vi "Move XYZ.vi"(0 "PID Gains In":T1={"X PID"={"proportional gain (Kc)"=0.03, "integral time (Ti, min)"=0.0, "derivative time (Td, min)"=0.0}, "Y PID"={"proportional gain (Kc)"=0.03, "integral time (Ti, min)"=0.0, "derivative time (Td, min)"=0.0}, "Z PID"={"proportional gain (Kc)"=0.035, "integral time (Ti, min)"=0.0, "derivative time (Td, min)"=0.0}} {"Z PID"."derivative time (Td, min)" format="%.3f"; "Z PID"."integral time (Ti, min)" format="%.3f"; "Z PID"."proportional gain (Kc)" format="%.3f"; "Y PID"."derivative time (Td, min)" format="%.3f"; "Y PID"."integral time (Ti, min)" format="%.3f"; "Y PID"."proportional gain (Kc)" format="%.3f"; "X PID"."derivative time (Td, min)" format="%.3f"; "X PID"."integral time (Ti, min)" format="%.3f"; "X PID"."proportional gain (Kc)" format="%.3f"}, 5 "Y Target":dbl, 6 "X Target":dbl, 10 "Max Time":dbl=90.0, 11 "Gyro Target":dbl=-180.0, 12 "Movement":dbl=3.0, 14 "X Output Range":cluster{"output high":dbl, "output low":dbl}={"output high"=0.8, "output low"=-0.8}, 15 "X Stop Threshold":dbl=5.0, 16 "Y Output Range":cluster{"output high":dbl, "output low":dbl}={"output high"=0.8, "output low"=-0.8}, 17 "Y Stop Threshold":dbl=5.0, 18 "Z Output Range":cluster{"output high":dbl, "output low":dbl}={"output high"=0.8, "output low"=-0.8}, 19 "Z  Stop Threshold":dbl=8.0) -> ()   [LabVIEW 2018]
uses:
  Robot Global Data.vi
  SubSystems/Drive Train/Drive Train Global.vi
  SubSystems/Hatch Panel Intake/Hatch Panel Intake Global.vi
  SubSystems/Lift/Lift Global.vi
  <vilib>/addons/control/pid/pid.llb/PID (DBL).vi
  <vilib>/addons/control/pid/NI_PID_pid.lvlib
panel:
  in  "Minimum Time":u32=500
  in  "Settle Time":u32=2000
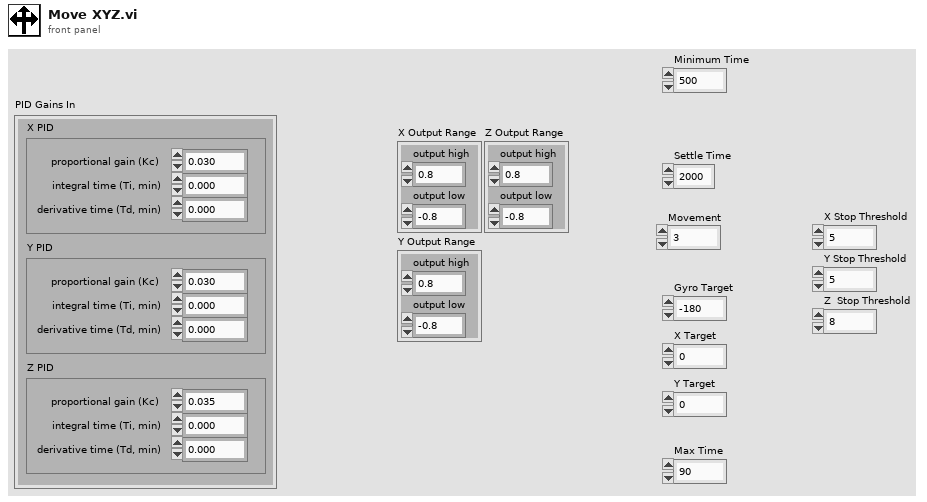
[diagram p1: front panel]
types:
  T1 = cluster{"X PID":cluster{"proportional gain (Kc)":dbl, "integral time (Ti, min)":dbl, "derivative time (Td, min)":dbl}, "Y PID":cluster{"proportional gain (Kc)":dbl, "integral time (Ti, min)":dbl, "derivative time (Td, min)":dbl}, "Z PID":cluster{"proportional gain (Kc)":dbl, "integral time (Ti, min)":dbl, "derivative time (Td, min)":dbl}}
  T2 = cluster{"proportional gain (Kc)":dbl, "integral time (Ti, min)":dbl, "derivative time (Td, min)":dbl}
  T3 = cluster{"Rollover":dbl, "Yaw":dbl, "Cont Yaw":dbl}
  T4 = cluster{"offsetAngle H":dbl, "offsetAngle V":dbl, "area":dbl, "skew":dbl, "validTarget":dbl, "latency":dbl}
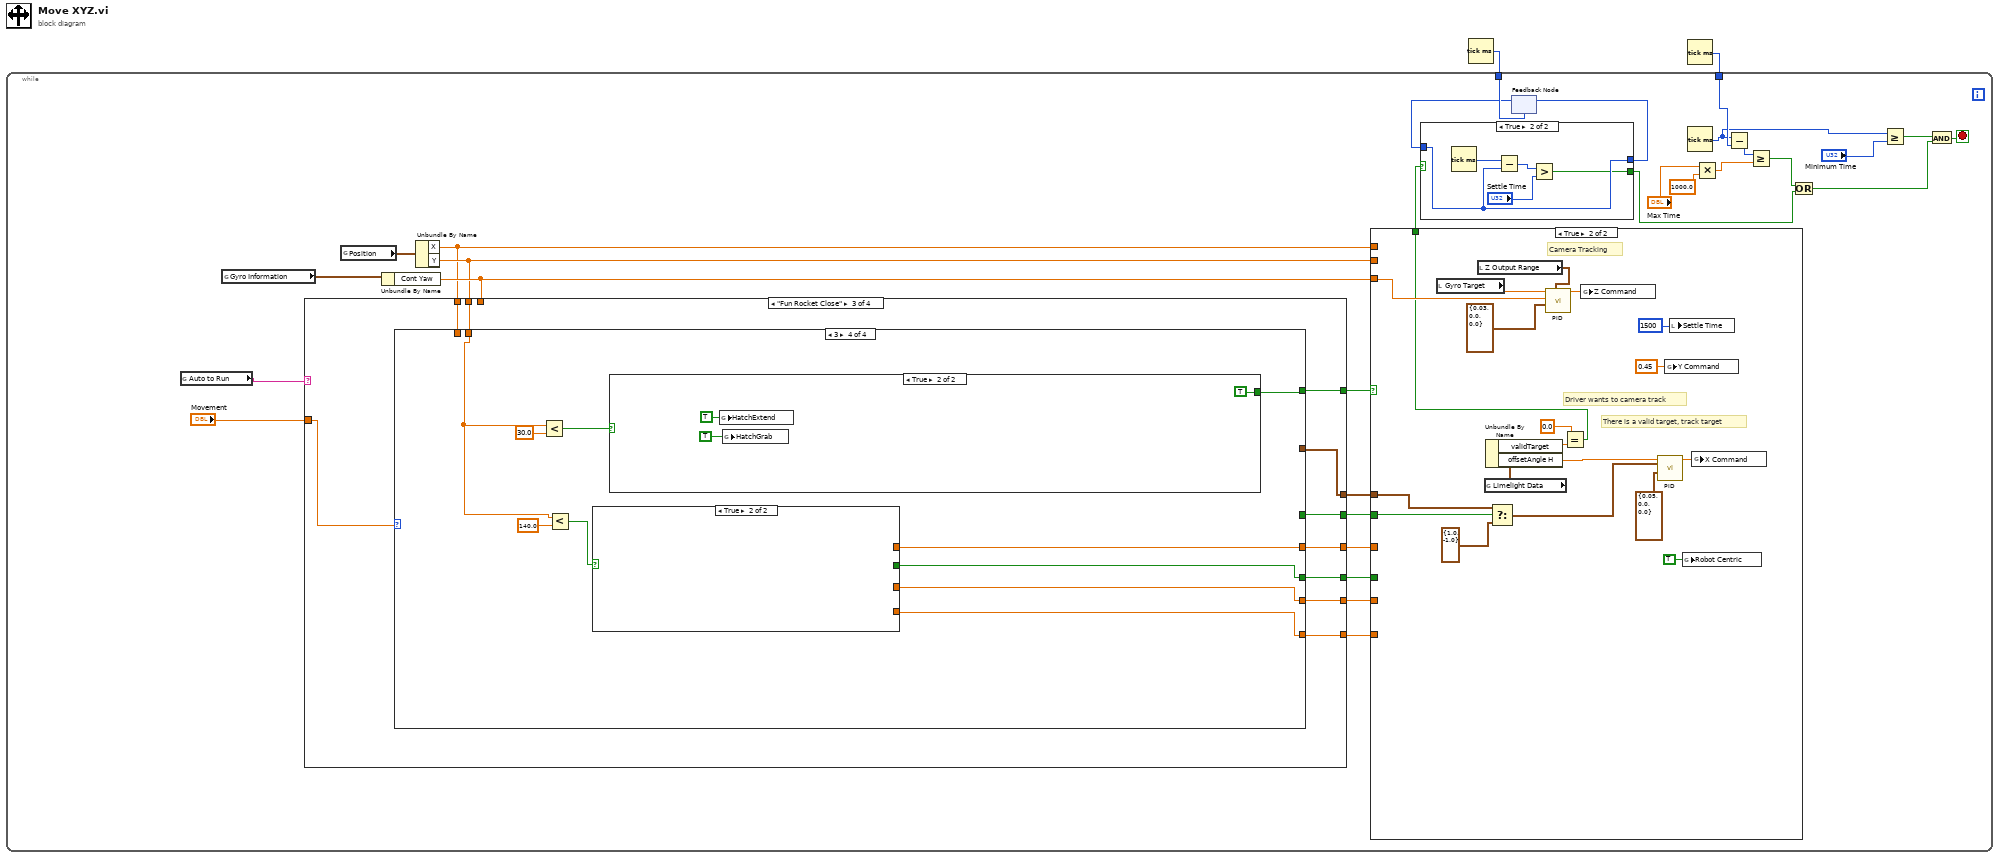
[diagram p0: block diagram]
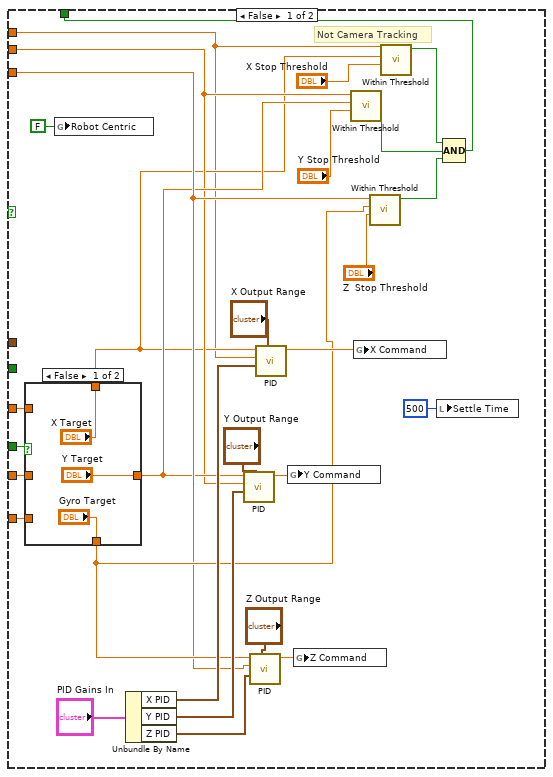
[diagram p2: hidden frame]
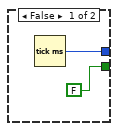
[diagram p4: hidden frame]
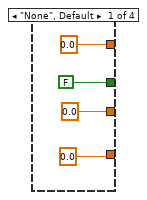
[diagram p5: hidden frame]
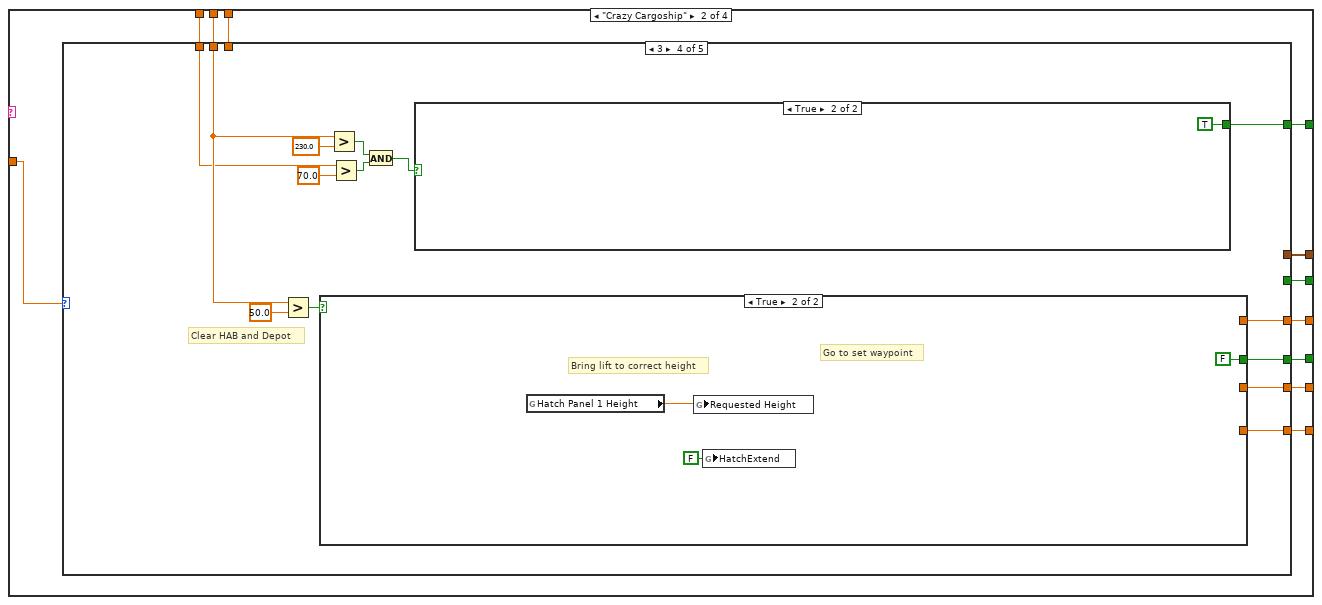
[diagram p6: hidden frame]
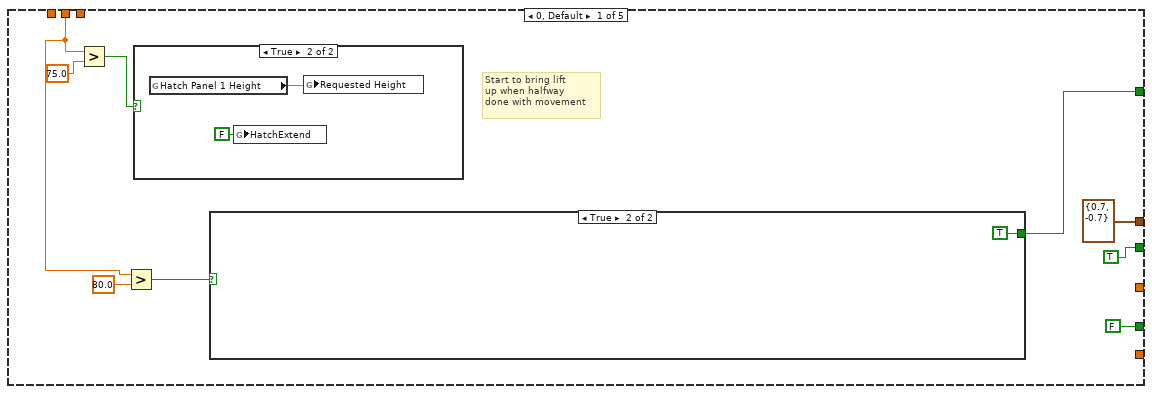
[diagram p7: hidden frame]
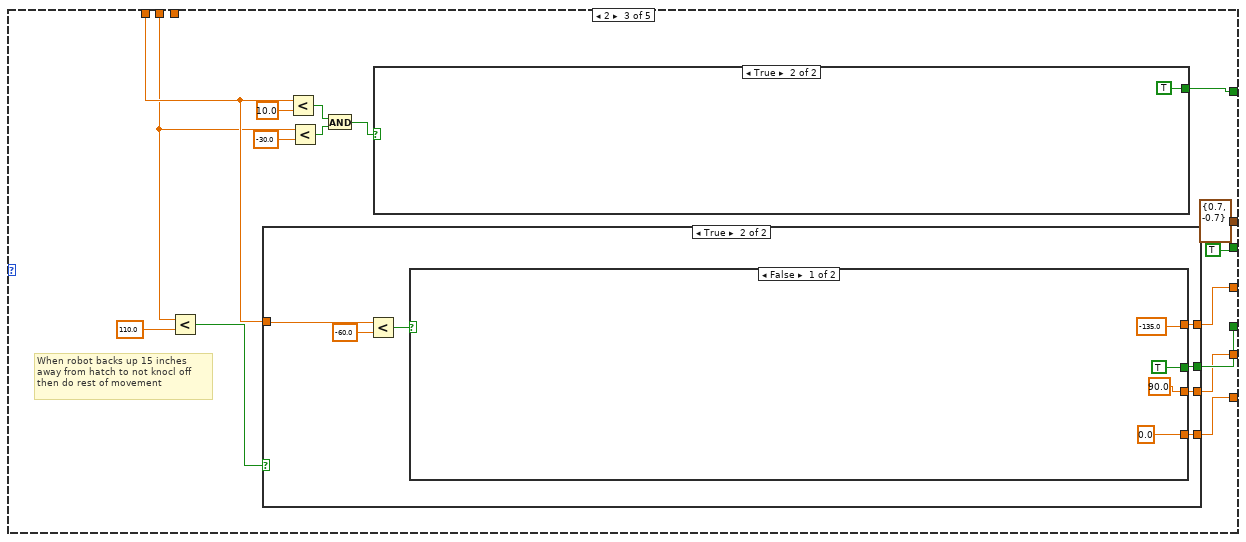
[diagram p11: hidden frame]
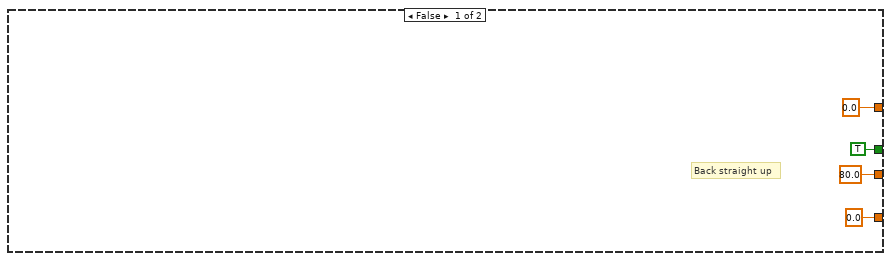
[diagram p13: hidden frame]
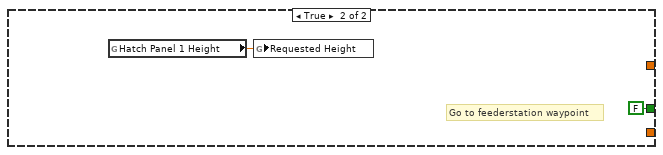
[diagram p14: hidden frame]
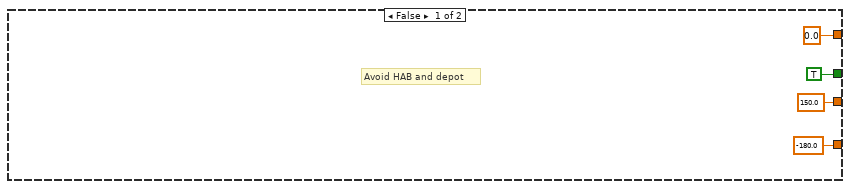
[diagram p16: hidden frame]
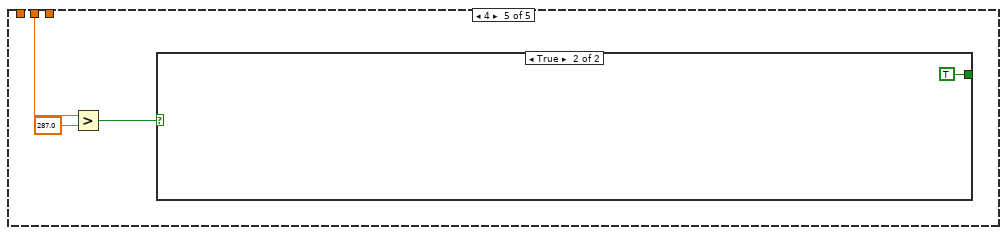
[diagram p17: hidden frame]
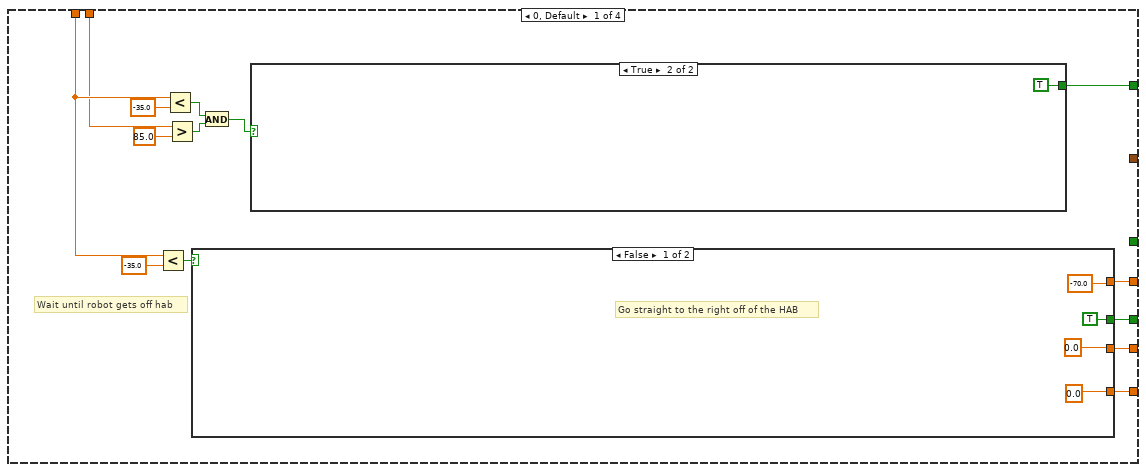
[diagram p19: hidden frame]
diagram:
  n1 = Tick Count (ms)() -> (millisecond timer value=w2:u32)
  n2 = Tick Count (ms)() -> (millisecond timer value=w1:u32)
  n3 = while {
    tunnel: w2 -> [w26]
    tunnel: w1 -> [w11]
    stop <- w10 stop-if-true
    n4 = global read "Robot Global Data.vi" "Auto to Run"() -> (w23:string)
    n5 = global read "Drive Train Global.vi" "Gyro Information"() -> (w20:T3)
    n6 = global read "Drive Train Global.vi" "Position"() -> (w22:cluster{"X":dbl, "Y":dbl})
    n7 = Unbundle By Name(w20) -> ("Cont Yaw"=w18:dbl)
    n8 = Unbundle By Name(w22) -> ("X"=w16:dbl, "Y"=w17:dbl)
    n9 = case shown="\"Fun Rocket Close\"" w23 {
      tunnel: [0.0 w103 w186 w268] -> w32
      tunnel: [0.0 w102 w185 w267] -> w31
      tunnel: [0.0 w101 w184 w266] -> w30
      tunnel: w17 -> [_ w107 w189 w271]
      tunnel: [FALSE w106 w187 w269] -> w29
      tunnel: w16 -> [_ w104 w188 w270]
      tunnel: "Movement" -> [_ w108 w190 w272]
      tunnel: w18 -> [_ w105 _ w264]
      tunnel: [_ w100 w183 w265] -> w5
      tunnel: [_ w98 w181 _] -> w4
      tunnel: [_ w99 w182 _] -> w3
      frame "None", Default {
      }
      frame "Crazy Cargoship" {
        n10 = case shown="3" w108 {
          tunnel: w107 -> [w111 _ w123 w156 w177]
          tunnel: [FALSE _ w134 w168 _] -> w106
          tunnel: w105 -> [_ _ _ _ _]
          tunnel: w104 -> [_ _ w124 w155 _]
          tunnel: [_ _ w133 w165 _] -> w103
          tunnel: [_ _ w132 w164 _] -> w102
          tunnel: [_ _ w131 w163 _] -> w101
          tunnel: [w113 _ w125 w157 _] -> w100
          tunnel: [TRUE ("Robot Centric") _ TRUE ("Robot Centric") _ _] -> w99
          tunnel: [cluster{"output high":dbl, "output low":dbl} {"output high"=0.7, "output low"=-0.7} ("output range") _ cluster{"output high":dbl, "output low":dbl} {"output high"=0.7, "output low"=-0.7} ("output range") _ _] -> w98
          frame 0, Default {
            # "Start to bring lift\nup when halfway\ndone with movement"
            n11 = Greater?(x=w111, y=75.0) -> (0:w116:bool)
            n12 = Greater?(x=w111, y=80.0) -> (0:w112:bool)
            n13 = case shown="True" w116 {
              frame False {
              }
              frame True {
                n14 = global read "Lift Global.vi" "Hatch Panel 1 Height"() -> (w120:dbl)
                n15 = global write "Hatch Panel Intake Global.vi" "HatchExtend"(FALSE ("HatchGrab")) -> ()
                n16 = global write "Lift Global.vi" "Requested Height"(w120) -> ()
              }
            }
            n17 = case shown="True" w112 {
              tunnel: [_ TRUE] -> w113
              frame False {
              }
              frame True {
              }
            }
          }
          frame 1 {
          }
          frame 2 {
            # "When robot backs up 15 inches\naway from hatch to not knocl off\nthen do rest of movement"
            n18 = Less?(x=w123, y=110.0) -> (x < y?=w136:bool)
            n19 = case shown="True" w136 {
              tunnel: [TRUE w148] -> w134
              tunnel: [0.0 w144] -> w133
              tunnel: [80.0 w143] -> w132
              tunnel: [0.0 w142] -> w131
              tunnel: w124 -> [_ w145]
              frame False {
                # "Back straight up"
              }
              frame True {
                n20 = Less?(x=w145, y=-60.0) -> (x < y?=w146:bool)
                n21 = case shown="False" w146 {
                  tunnel: [TRUE FALSE] -> w148
                  tunnel: [-135.0 _] -> w144
                  tunnel: [90.0 _] -> w143
                  tunnel: [0.0 _] -> w142
                  frame False {
                  }
                  frame True {
                    # "Go to feederstation waypoint"
                    n22 = global read "Lift Global.vi" "Hatch Panel 1 Height"() -> (w153:dbl)
                    n23 = global write "Lift Global.vi" "Requested Height"(w153) -> ()
                  }
                }
              }
            }
            n24 = Less?(x=w124, y=10.0) -> (x < y?=w128:bool)
            n25 = Less?(x=w123, y=-30.0) -> (x < y?=w127:bool)
            n26 = And(x=w128, y=w127) -> (x .and. y?=w126:bool)
            n27 = case shown="True" w126 {
              tunnel: [_ TRUE] -> w125
              frame False {
              }
              frame True {
              }
            }
          }
          frame 3 {
            # "Clear HAB and Depot"
            n28 = Greater?(x=w156, y=50.0) -> (0:w167:bool)
            n29 = case shown="True" w167 {
              tunnel: [TRUE FALSE] -> w168
              tunnel: [0.0 _] -> w165
              tunnel: [150.0 _] -> w164
              tunnel: [-180.0 _] -> w163
              frame False {
                # "Avoid HAB and depot"
              }
              frame True {
                # "Bring lift to correct height"
                # "Go to set waypoint"
                n30 = global read "Lift Global.vi" "Hatch Panel 1 Height"() -> (w175:dbl)
                n31 = global write "Lift Global.vi" "Requested Height"(w175) -> ()
                n32 = global write "Hatch Panel Intake Global.vi" "HatchExtend"(FALSE ("HatchGrab")) -> ()
              }
            }
            n33 = Greater?(x=w156, y=230.0) -> (0:w160:bool)
            n34 = Greater?(x=w155, y=70.0) -> (0:w159:bool)
            n35 = And(x=w160, y=w159) -> (x .and. y?=w158:bool)
            n36 = case shown="True" w158 {
              tunnel: [_ TRUE] -> w157
              frame False {
              }
              frame True {
              }
            }
          }
          frame 4 {
            n37 = Greater?(x=w177, y=287.0) -> (0:w178:bool)
            n38 = case shown="True" w178 {
              tunnel: [_ TRUE] -> _
              frame False {
              }
              frame True {
              }
            }
          }
        }
      }
      frame "Fun Rocket Close" {
        n39 = case shown="3" w190 {
          tunnel: w189 -> [w197 w212 w231 w252]
          tunnel: w188 -> [w198 w217 _ _]
          tunnel: [w202 _ w229 w247] -> w187
          tunnel: [w201 _ w230 w250] -> w186
          tunnel: [w200 _ w228 w249] -> w185
          tunnel: [w199 _ w227 w248] -> w184
          tunnel: [w191 w218 w237 w255] -> w183
          tunnel: [_ _ w235 _] -> w182
          tunnel: [_ _ w234 _] -> w181
          frame 0, Default {
            # "Wait until robot gets off hab"
            n40 = Less?(x=w198, y=-35.0) -> (x < y?=w204:bool)
            n41 = Less?(x=w198, y=-35.0) -> (x < y?=w194:bool)
            n42 = Greater?(x=w197, y=85.0) -> (0:w193:bool)
            n43 = case shown="False" w204 {
              tunnel: [TRUE FALSE] -> w202
              tunnel: [-70.0 _] -> w201
              tunnel: [0.0 _] -> w200
              tunnel: [0.0 _] -> w199
              frame False {
                # "Go straight to the right off of the HAB"
              }
              frame True {
                # "Bring the lift up to the correct level because its slow"
                # "Robot off of HAB, go to the rocket"
                n44 = global read "Lift Global.vi" "Hatch Panel 2 Height"() -> (w210:dbl)
                n45 = global write "Lift Global.vi" "Requested Height"(w210) -> ()
              }
            }
            n46 = And(x=w194, y=w193) -> (x .and. y?=w192:bool)
            n47 = case shown="True" w192 {
              tunnel: [_ TRUE] -> w191
              frame False {
              }
              frame True {
              }
            }
          }
          frame 1 {
            n48 = Less?(x=w212, y=-17.0) -> (x < y?=w221:bool)
            n49 = Less?(x=w217, y=-90.0) -> (x < y?=w220:bool)
            n50 = Less?(x=w212, y=0.0) -> (x < y?=w215:bool)
            n51 = Less?(x=w212, y=-5.0) -> (x < y?=w214:bool)
            n52 = And(x=w221, y=w220) -> (x .and. y?=w219:bool)
            n53 = case shown="True" w215 {
              frame False {
              }
              frame True {
                n54 = global write "Hatch Panel Intake Global.vi" "HatchExtend"(TRUE ("HatchExtend")) -> ()
              }
            }
            n55 = case shown="True" w214 {
              frame False {
              }
              frame True {
                n56 = global write "Hatch Panel Intake Global.vi" "HatchGrab"(TRUE ("HatchExtend")) -> ()
              }
            }
            n57 = case shown="True" w219 {
              tunnel: [_ TRUE] -> w218
              frame False {
              }
              frame True {
              }
            }
          }
          frame 2 {
            # "back up then turn"
            n58 = Greater?(x=w231, y=150.0) -> (0:w236:bool)
            n59 = Greater?(x=w231, y=40.0) -> (0:w232:bool)
            n60 = case shown="True" w236 {
              tunnel: [_ TRUE] -> w237
              tunnel: [_ TRUE] -> w235
              tunnel: [_ cluster{"output high":dbl, "output low":dbl} {"output high"=0.6, "output low"=-0.6} ("output range")] -> w234
              frame False {
              }
              frame True {
              }
            }
            n61 = case shown="False" w232 {
              tunnel: [0.0 _] -> w230
              tunnel: [TRUE FALSE] -> w229
              tunnel: [200.0 _] -> w228
              tunnel: [-180.0 _] -> w227
              frame False {
              }
              frame True {
              }
            }
          }
          frame 3 {
            n62 = Less?(x=w252, y=30.0) -> (x < y?=w254:bool)
            n63 = Less?(x=w252, y=140.0) -> (x < y?=w251:bool)
            n64 = case shown="True" w251 {
              tunnel: [0.0 _] -> w250
              tunnel: [100.0 _] -> w249
              tunnel: [-30.0 _] -> w248
              tunnel: [TRUE _] -> w247
              frame False {
              }
              frame True {
              }
            }
            n65 = case shown="True" w254 {
              tunnel: [_ TRUE] -> w255
              frame False {
              }
              frame True {
                n66 = global write "Hatch Panel Intake Global.vi" "HatchExtend"(TRUE ("HatchExtend")) -> ()
                n67 = global write "Hatch Panel Intake Global.vi" "HatchGrab"(TRUE ("HatchExtend")) -> ()
              }
            }
          }
        }
      }
      frame "Fun Rocket Far" {
        n68 = case shown="2" w272 {
          tunnel: w271 -> [w275 w309 w328 w344]
          tunnel: w270 -> [w274 w307 _ _]
          tunnel: [w279 w305 w333 w339] -> w269
          tunnel: [w278 w306 w332 w342] -> w268
          tunnel: [w277 w304 w331 w341] -> w267
          tunnel: [w276 w303 w330 w340] -> w266
          tunnel: [w273 w312 _ w347] -> w265
          tunnel: w264 -> [_ _ _ _]
          frame 0, Default {
            # "Wait until robot gets off hab"
            n69 = Greater?(x=w275, y=160.0) -> (0:w281:bool)
            n70 = case shown="True" w281 {
              tunnel: [TRUE w294] -> w279
              tunnel: [-10.0 w292] -> w278
              tunnel: [170.0 w291] -> w277
              tunnel: [0.0 w290] -> w276
              tunnel: w274 -> [_ w287]
              tunnel: [_ w286] -> w273
              frame False {
              }
              frame True {
                # "Bring the lift up to the correct level because its slow"
                n71 = global read "Lift Global.vi" "Hatch Panel 2 Height"() -> (w293:dbl)
                n72 = global write "Lift Global.vi" "Requested Height"(w293) -> ()
                n73 = Less?(x=w287, y=-60.0) -> (x < y?=w288:bool)
                n74 = case shown="False" w288 {
                  tunnel: [TRUE FALSE] -> w294
                  tunnel: [-100.0 ("y") _] -> w292
                  tunnel: [195.0 ("y") _] -> w291
                  tunnel: [-150.0 ("y") _] -> w290
                  tunnel: [_ TRUE] -> w286
                  frame False {
                  }
                  frame True {
                  }
                }
              }
            }
          }
          frame 1 {
            n75 = Less?(x=w309, y=-30.0) -> (x < y?=w315:bool)
            n76 = Greater?(x=w307, y=65.0) -> (0:w314:bool)
            n77 = Less?(x=w309, y=0.0) -> (x < y?=w310:bool)
            n78 = And(x=w315, y=w314) -> (x .and. y?=w313:bool)
            n79 = case shown="True" w310 {
              frame False {
              }
              frame True {
                n80 = global write "Hatch Panel Intake Global.vi" "HatchExtend"(TRUE ("HatchExtend")) -> ()
                n81 = global write "Hatch Panel Intake Global.vi" "HatchGrab"(TRUE ("HatchExtend")) -> ()
              }
            }
            n82 = Greater?(x=w307, y=-40.0) -> (0:w301:bool)
            n83 = case shown="False" w313 {
              tunnel: [FALSE TRUE] -> w312
              frame False {
              }
              frame True {
              }
            }
            n84 = call "Flip Flop.vi"("Line 1"=w301) -> ("Switch"=w302:bool)  [unwired: 10 in]
            n85 = case shown="True" w302 {
              tunnel: [_ -30.0 ("y")] -> w306
              tunnel: [FALSE TRUE] -> w305
              tunnel: [_ 190.0 ("y")] -> w304
              tunnel: [_ -150.0 ("y")] -> w303
              frame False {
              }
              frame True {
              }
            }
          }
          frame 2 {
            n86 = Less?(x=w328, y=30.0) -> (x < y?=w329:bool)
            n87 = case shown="False" w329 {
              tunnel: [TRUE FALSE] -> w333
              tunnel: [-30.0 _] -> w332
              tunnel: [100.0 _] -> w331
              tunnel: [-180.0 _] -> w330
              frame False {
              }
              frame True {
              }
            }
          }
          frame 3 {
            n88 = Less?(x=w344, y=30.0) -> (x < y?=w346:bool)
            n89 = Less?(x=w344, y=140.0) -> (x < y?=w343:bool)
            n90 = case shown="False" w343 {
              tunnel: [0.0 _] -> w342
              tunnel: [100.0 _] -> w341
              tunnel: [-30.0 _] -> w340
              tunnel: [TRUE _] -> w339
              frame False {
              }
              frame True {
              }
            }
            n91 = case shown="True" w346 {
              tunnel: [_ TRUE] -> w347
              frame False {
              }
              frame True {
              }
            }
          }
        }
      }
    }
    n92 = case shown="True" w5 {
      tunnel: w32 -> [w54 _]
      tunnel: w31 -> [w53 _]
      tunnel: w30 -> [w52 _]
      tunnel: w29 -> [w51 _]
      tunnel: [w35 w73] -> w19
      tunnel: w18 -> [w45 w77]
      tunnel: w17 -> [w41 _]
      tunnel: w16 -> [w37 _]
      tunnel: w4 -> [_ w70]
      tunnel: w3 -> [_ w69]
      frame False {
        # "Not Camera Tracking"
        n93 = case shown="False" w51 {
          tunnel: ["X Target" w67] -> w38
          tunnel: ["Y Target" w66] -> w42
          tunnel: ["Gyro Target" w65] -> w46
          tunnel: w54 -> [_ w67]
          tunnel: w53 -> [_ w66]
          tunnel: w52 -> [_ w65]
          frame False {
          }
          frame True {
          }
        }
        n94 = global write "Drive Train Global.vi" "Robot Centric"(FALSE ("Robot Centric")) -> ()
        n95 = Unbundle By Name("PID Gains In") -> ("X PID"=w59:T2, "Y PID"=w58:T2, "Z PID"=w57:T2)
        n96 = call-poly <vilib>:"PID.vi"("output range"="Y Output Range", "PID gains"=w58, "process variable"=w41, "setpoint"=w42) -> ("output"=w48:dbl)  [unwired: 6 in, 1 out]
        n97 = call-poly <vilib>:"PID.vi"("output range"="Z Output Range", "PID gains"=w57, "process variable"=w45, "setpoint"=w46) -> ("output"=w49:dbl)  [unwired: 6 in, 1 out]
        n98 = call-poly <vilib>:"PID.vi"("output range"="X Output Range", "PID gains"=w59, "process variable"=w37, "setpoint"=w38) -> ("output"=w50:dbl)  [unwired: 6 in, 1 out]
        n99 = global write "Drive Train Global.vi" "Y Command"(w48) -> ()
        n100 = global write "Drive Train Global.vi" "Z Command"(w49) -> ()
        n101 = call "Within Threshold.vi"("Threshold"="Y Stop Threshold", "Center"=w42, "Value"=w41) -> ("Within Threshold?"=w43:bool)  [unwired: 8 in]
        n102 = global write "Drive Train Global.vi" "X Command"(w50) -> ()
        n103 = call "Within Threshold.vi"("Threshold"="Z  Stop Threshold", "Center"=w46, "Value"=w45) -> ("Within Threshold?"=w47:bool)  [unwired: 8 in]
        n104 = call "Within Threshold.vi"("Threshold"="X Stop Threshold", "Center"=w38, "Value"=w37) -> ("Within Threshold?"=w39:bool)  [unwired: 8 in]
        n105 = local write "Settle Time"(u32 500 ("Settle Time")) -> ()
        n106 = Compound Arithmetic op=AND(w39, w43, w47) -> (w35:bool)
      }
      frame True {
        # "There is a valid target, track target"
        # "Driver wants to camera track"
        # "Camera Tracking"
        n107 = local read "Gyro Target"() -> (w78:dbl)
        n108 = local read "Z Output Range"() -> (w79:cluster{"output high":dbl, "output low":dbl})
        n109 = global read "Robot Global Data.vi" "Limelight Data"() -> (w84:T4)
        n110 = Unbundle By Name(w84) -> ("validTarget"=w75:dbl, "offsetAngle H"=w83:dbl)
        n111 = Select(t=w70, s=w69, f=cluster{"output high":dbl, "output low":dbl} {"output high"=1.0, "output low"=-1.0} ("output range")) -> (s? t:f=w71:cluster{"output high":dbl, "output low":dbl})
        n112 = call-poly <vilib>:"PID.vi"("output range"=w79, "PID gains"=T2 {"proportional gain (Kc)"=0.03, "integral time (Ti, min)"=0.0, "derivative time (Td, min)"=0.0}, "process variable"=w77, "setpoint"=w78) -> ("output"=w80:dbl)  [unwired: 6 in, 1 out]
        n113 = Equal?(x=0.0, y=w75) -> (x = y?=w73:bool)
        n114 = global write "Drive Train Global.vi" "Z Command"(w80) -> ()
        n115 = call-poly <vilib>:"PID.vi"("output range"=w71, "PID gains"=T2 {"proportional gain (Kc)"=0.05, "integral time (Ti, min)"=0.0, "derivative time (Td, min)"=0.0} ("Camera Tracking"), "setpoint"=w83) -> ("output"=w85:dbl)  [unwired: 7 in, 1 out]
        n116 = global write "Drive Train Global.vi" "Y Command"(0.45 ("Y Command")) -> ()
        n117 = local write "Settle Time"(u32 1500 ("Settle Time")) -> ()
        n118 = global write "Drive Train Global.vi" "Robot Centric"(TRUE ("Robot Centric")) -> ()
        n119 = global write "Drive Train Global.vi" "X Command"(w85) -> ()
      }
    }
    n120 = feedback #1(w26) -> (w25:u32)
    n121 = case shown="True" w19 {
      tunnel: [w88 w91] -> w27
      tunnel: w25 -> [_ w91]
      tunnel: [FALSE w90] -> w24
      frame False {
        n122 = Tick Count (ms)() -> (millisecond timer value=w88:u32)
      }
      frame True {
        n123 = Tick Count (ms)() -> (millisecond timer value=w93:u32)
        n124 = Subtract(x=w93, y=w91) -> (x-y=w92:u32)
        n125 = Greater?(x=w92, y="Settle Time") -> (0:w90:bool)
      }
    }
    n126 = feedback-in #1(w27) -> ()
    n127 = Tick Count (ms)() -> (millisecond timer value=w9:u32)
    n128 = Multiply(x="Max Time", y=1000.0) -> (x*y=w14:dbl)
    n129 = Subtract(x=w9, y=w11) -> (x-y=w15:u32)
    n130 = Greater Or Equal?(x=w15, y=w14) -> (x >= y?=w28:bool)
    n131 = Or(x=w28, y=w24) -> (x .or. y?=w6:bool)
    n132 = Greater Or Equal?(x=w9, y="Minimum Time") -> (x >= y?=w7:bool)
    n133 = And(x=w7, y=w6) -> (x .and. y?=w10:bool)
  }
